vi "Close Connection.vi"(2 "error in (no error)":errorcluster, 3 "Database.lvlib:Data Store.lvclass":refnum<class "Data Store.lvclass">) -> (0 "error out":errorcluster)   [LabVIEW 2011, in "Database.lvlib" / "Data Store.lvclass"]
uses:
  Data Store.lvclass
  Data Store.lvclass/Data Store.ctl
  <vilib>/addons/database/NI_Database_API.lvlib
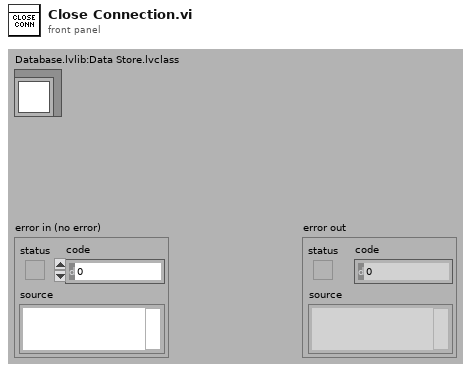
[diagram p1: front panel]
types:
  T1 = typedef "NI_Database_API.lvlib/Conn ObjectReference.ctl" = refnum<k1>
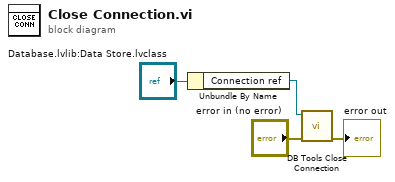
[diagram p0: block diagram]
diagram:
  n1 = Unbundle By Name("Database.lvlib:Data Store.lvclass") -> ("Connection ref"=w1:T1)
  n2 = call <vilib>:"DB Tools Close Connection.vi"("error in (no error)"="error in (no error)", "connection reference"=w1) -> ("error out"=→"error out":errorcluster)  [unwired: 5 in]
